vi "nanoindentation_v1.vi"() -> ()   [LabVIEW 2014]
uses:
  <userlib>/Nanonis Prog Interface V5/Nanonis Prog Interface.lvlib
panel:
  in  "Gain":u16(ring)=11 items=["HS 10^5", "HS 10^6", "HS 10^7", "HS 10^8", "HS 10^9", "HS 10^10", "HS 10^11", "LN 10^3", "LN 10^4", "LN 10^5", "LN 10^6", "LN 10^7", "LN 10^8", "LN 10^9"]
  in  "Bias (V)":sgl=0.02 format="%#_5p"
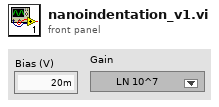
[diagram p1: front panel]
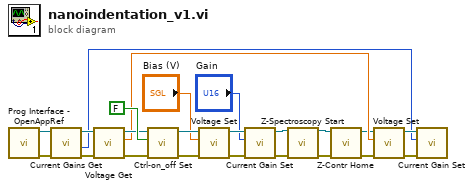
[diagram p0: block diagram]
diagram:
  n1 = call <userlib>:"Prog Interface - OpenAppRef.vi"() -> ("Error out"=w6:errorcluster, "Application reference"=w7:refnum<vi>)  [unwired: 6 in]
  n2 = call <userlib>:"Current Gains Get.vi"("Error in (no error)"=w6, "Application ref in"=w7) -> ("Error out"=w4:errorcluster, "Selected Gain"=w1:u16, "Application ref out"=w5:refnum<vi>)  [unwired: 6 in, 1 out]
  n3 = call <userlib>:"Voltage Get.vi"("error in (no error)"=w4, "Application ref in"=w5) -> ("error out"=w13:errorcluster, "Bias (V)"=w12:sgl, "Application ref out"=w14:refnum<vi>)  [unwired: 7 in]
  n4 = call <userlib>:"Ctrl-on_off Set.vi"("error in (no error)"=w13, "Z Controller ON/OFF"=FALSE, "Application ref in"=w14) -> ("error out"=w22:errorcluster, "Application ref out"=w21:refnum<vi>)  [unwired: 7 in]
  n5 = call <userlib>:"Voltage Set.vi"("Error in (no error)"=w22, "Bias (V)"="Bias (V)", "Application ref in"=w21) -> ("Error out"=w19:errorcluster, "Application ref out"=w18:refnum<vi>)  [unwired: 7 in]
  n6 = call <userlib>:"Current Gain Set.vi"("Error in (no error)"=w19, "Gain index"="Gain", "Application ref in"=w18) -> ("Error out"=w15:errorcluster, "Application ref out"=w16:refnum<vi>)  [unwired: 7 in]
  n7 = call <userlib>:"Z-Spectroscopy Start.vi"("Application ref in"=w16, "error in (no error)"=w15) -> ("Application ref out"=w10:refnum<vi>, "error out"=w11:errorcluster)  [unwired: 9 in, 3 out]
  n8 = call <userlib>:"Z-Contr Home.vi"("Error in (no error)"=w11, "Application ref in"=w10) -> ("Error out"=w9:errorcluster, "Application ref out"=w8:refnum<vi>)  [unwired: 8 in]
  n9 = call <userlib>:"Voltage Set.vi"("Error in (no error)"=w9, "Bias (V)"=w12, "Application ref in"=w8) -> ("Error out"=w3:errorcluster, "Application ref out"=w2:refnum<vi>)  [unwired: 7 in]
  n10 = call <userlib>:"Current Gain Set.vi"("Error in (no error)"=w3, "Gain index"=w1, "Application ref in"=w2) -> ()  [unwired: 7 in, 2 out]
